vi "Advanced Example.vi"() -> ()   [LabVIEW 2010]
doc: "This VI demonstrates the advanced index-based functionality."
uses:
  Type Defs/Data Types.ctl
  Type Defs/File Format.ctl
  Type Defs/Single Tag.ctl
  Type Defs/Tag Grouping set.ctl
  DataTypes/Double_Get Index.vi
  DataTypes/Double_Read Index.vi
  DataTypes/Single_Read Index Set.vi
  Type to Enum.vi
  DataTypes/Double_Type To Enum.vi
  FGVs/Tag Memory.vi
  Memory Block.vi
  DataTypes/Double_Memory Block.vi
  DataTypes/Single_Memory Block.vi
  Current Value Table.lvlib
panel:
  out "Tag 4":sgl
  out "Tag 3":sgl
  out "error out":errorcluster
  out "Expected Error":errorcluster
  out "Tag 1":dbl
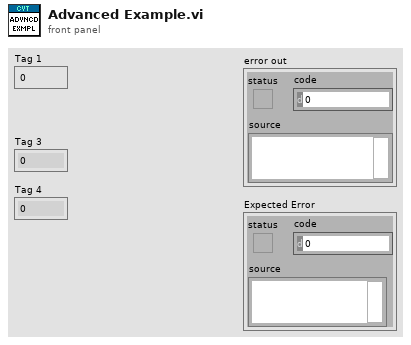
[diagram p1: front panel]
types:
  T1 = typedef "Current Value Table.lvlib/Data Types.ctl" = enum16{"Double", "Single", "I64", "I32", "I16", "I8", "U64", "U32", "U16", "U8", "String", "Boolean", "Array of U8", "Array of U16", "Array of U32", "Array of U64", "Array of I64", "Array of I32", "Array of I16", "Array of I8", "Array of Double", "Array of Single", "Array of Boolean", "Array of String"}
  T2 = typedef "Current Value Table.lvlib/File Format.ctl" = cluster{"Tags":T3[], "Group Listings":T4[]}
  T3 = typedef "Current Value Table.lvlib/Single Tag.ctl" = cluster{"Data Type":T1, "Name":string, "Value":string, "Description":string}
  T4 = typedef "Current Value Table.lvlib/Tag Grouping set.ctl" = cluster{"Group":string, "Tag Names":string[]}
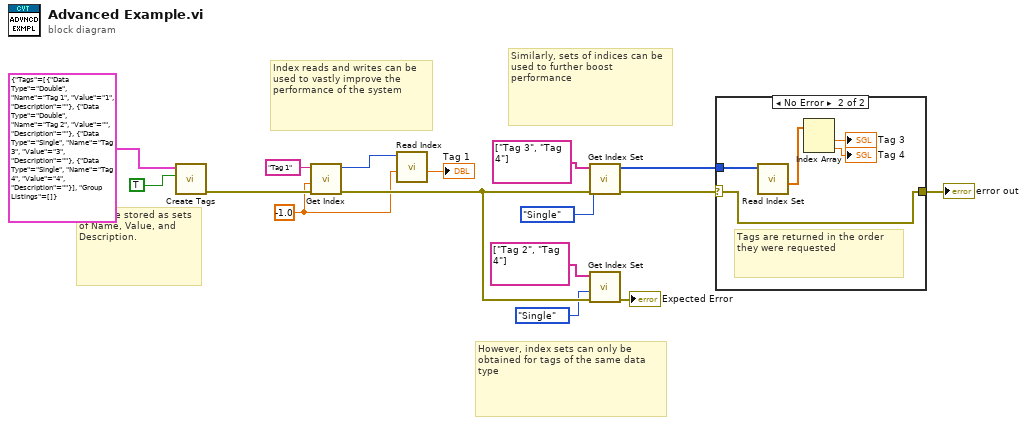
[diagram p0: block diagram]
diagram:
  w4 = -1.0 ("Default")
  # "However, index sets can only be obtained for tags of the same data type"
  # "Similarly, sets of indices can be used to further boost performance"
  # "Index reads and writes can be used to vastly improve the performance of the system"
  # "Tags are stored as sets of Name, Value, and Description."
  n1 = call "Create Tags.vi"("Clear Table? (F)"=TRUE ("Clear Engine?"), "CVT Tags to Create"=T2 {"Tags"=[{"Data Type"=enum."Double", "Name"="Tag 1", "Value"="1", "Description"=""}, {"Data Type"=enum."Double", "Name"="Tag 2", "Value"="", "Description"=""}, {"Data Type"=enum."Single", "Name"="Tag 3", "Value"="3", "Description"=""}, {"Data Type"=enum."Single", "Name"="Tag 4", "Value"="4", "Description"=""}], "Group Listings"=[]} ("CVT File Data")) -> ("error out"=w14:errorcluster)  [unwired: 9 in]
  n2 = call-poly "Get Index.vi"("error in (no error)"=w14, "Default"=w4, "Tag Name"="Tag 1") -> ("error out"=w8:errorcluster, "Index"=w12:i32)  [unwired: 7 in]
  n3 = call-poly "Read Index.vi"("Default"=w4, "Index"=w12) -> ("Value"=→"Tag 1":dbl)  [unwired: 9 in]
  n4 = call "Get Index Set.vi"("error in (no error)"=w8, "Expected Type"=Data_Types."Single", "Tag Names"=string[] ["Tag 3", "Tag 4"]) -> ("error out"=w1:errorcluster, "Tag References"=w6:i32[])  [unwired: 7 in]
  n5 = call "Get Index Set.vi"("error in (no error)"=w8, "Expected Type"=Data_Types."Single", "Tag Names"=string[] ["Tag 2", "Tag 4"]) -> ("error out"=→"Expected Error":errorcluster)  [unwired: 7 in, 1 out]
  n6 = case shown="No Error" w1 {
    selector: w1 -> [w17 w18]
    tunnel: w6 -> [_ w22]
    tunnel: [w17 w18] -> w5
    frame Error {
    }
    frame No Error {
      # "Tags are returned in the order they were requested"
      n7 = call-poly "Read Index Set.vi"("Indices"=w22) -> ("Values"=w21:sgl[])  [unwired: 10 in]
      n8 = Index Array(array=w21) -> (element #1=→"Tag 3":sgl, element #2=→"Tag 4":sgl)  [unwired: 2 in]
    }
  }
  "error out" <- w5
